vi "distance_sensor_model.vi"(10 "voltage_input":dbl) -> (2 "distance_output":dbl)   [LabVIEW 2020]
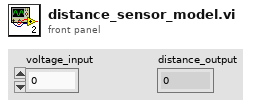
[diagram p1: front panel]
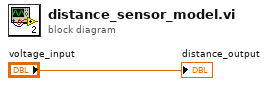
[diagram p0: block diagram]
diagram:
  "distance_output" <- "voltage_input"
